vi "3-4-2 gen random multi-data.vi"() -> (3 "output cluster":T1)   [LabVIEW 2020]
uses:
  <vilib>/numeric/Random Number (Range) DBL.vi
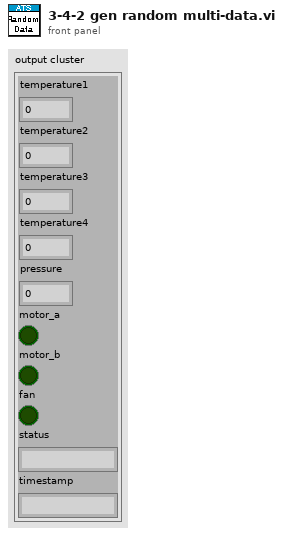
[diagram p1: front panel]
types:
  T1 = cluster{"temperature1":dbl, "temperature2":dbl, "temperature3":dbl, "temperature4":dbl, "pressure":dbl, "motor_a":bool, "motor_b":bool, "fan":bool, "status":string, "timestamp":string}
  T2 = cluster{"temperature1":dbl, "temperature2":dbl, "temperature3":dbl, "temperature4":dbl, "pressure":dbl, "motor_a":bool, "motor_b":bool, "motor_fan":bool, "status":string, "timestamp":string}
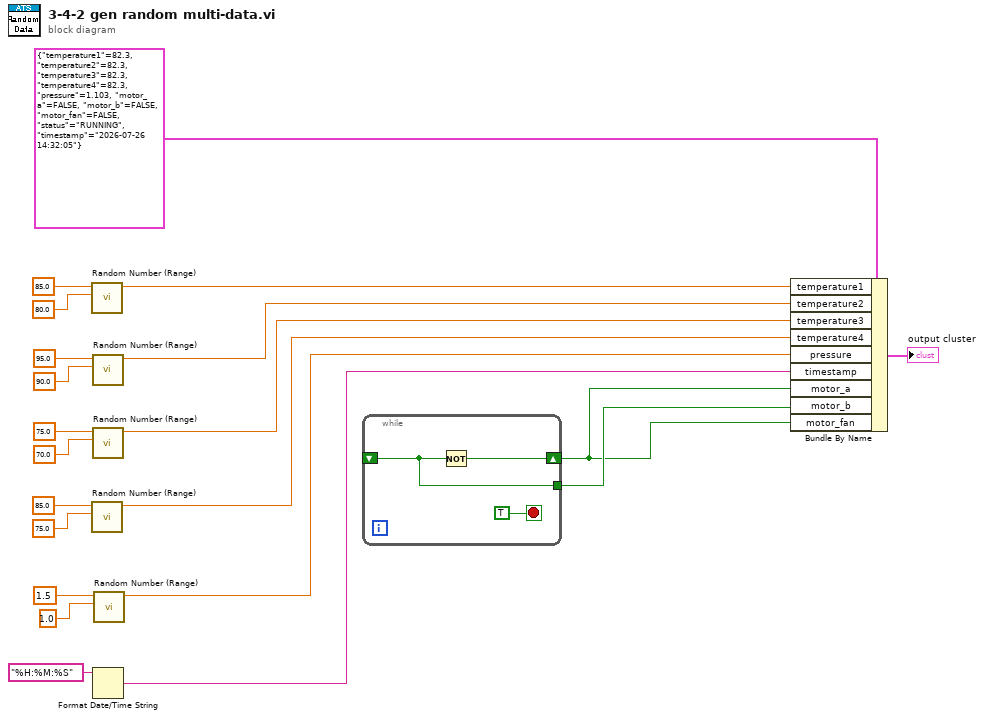
[diagram p0: block diagram]
diagram:
  n1 = call-poly <vilib>:"Random Number (Range).vi"("lower bound (0)"=80.0 ("upper bound (100)"), "upper bound (100)"=85.0) -> ("number"=w7:dbl)  [unwired: 9 in]
  n2 = call-poly <vilib>:"Random Number (Range).vi"("lower bound (0)"=75.0 ("upper bound (100)"), "upper bound (100)"=85.0) -> ("number"=w4:dbl)  [unwired: 9 in]
  n3 = call-poly <vilib>:"Random Number (Range).vi"("lower bound (0)"=90.0 ("upper bound (100)"), "upper bound (100)"=95.0) -> ("number"=w6:dbl)  [unwired: 9 in]
  n4 = call-poly <vilib>:"Random Number (Range).vi"("lower bound (0)"=70.0 ("upper bound (100)"), "upper bound (100)"=75.0) -> ("number"=w5:dbl)  [unwired: 9 in]
  n5 = Format Date/Time String(time format string (%c)="%H:%M:%S") -> (date/time string=w14:string)  [unwired: 2 in]
  n6 = call-poly <vilib>:"Random Number (Range).vi"("lower bound (0)"=1.0 ("upper bound (100)"), "upper bound (100)"=1.5) -> ("number"=w15:dbl)  [unwired: 9 in]
  n7 = while {
    shift-right: [w24] -> w1
    shift-left: _ -> [w22]
    tunnel: [w22] -> w2
    stop <- TRUE stop-if-true
    n8 = Not(x=w22) -> (.not. x?=w24:bool)
  }
  n9 = Bundle By Name(cluster=T2 {"temperature1"=82.3, "temperature2"=82.3, "temperature3"=82.3, "temperature4"=82.3, "pressure"=1.103, "motor_a"=FALSE, "motor_b"=FALSE, "motor_fan"=FALSE, "status"="RUNNING", "timestamp"="2026-07-26 14:32:05"} ("sensor_data"), "temperature1"=w7, "temperature2"=w6, "temperature3"=w5, "temperature4"=w4, "pressure"=w15, "timestamp"=w14, "motor_a"=w1, "motor_b"=w2, "motor_fan"=w1) -> (→"output cluster":T2)
